vi "Sondenmodell.GetRef.vi"(8 "Error In":errorcluster) -> (0 "Error out":errorcluster, 3 "Sondenmodell":refnum<data-value>)   [LabVIEW 2016, in "Sondenmodell.lvclass"]
uses:
  Sondenmodell.lvclass
  Package ResourceControl/ObjectHandler/ObjectHandler.GetObjectWType.ctl
  Package ResourceControl/ObjectHandler/ObjectHandler.ObjectWType.ctl
  Package ResourceControl/ObjectHandler/ObjectHandler.ObjectType.ctl
  Package ResourceControl/ObjectHandler/ObjectHandler.lvclass
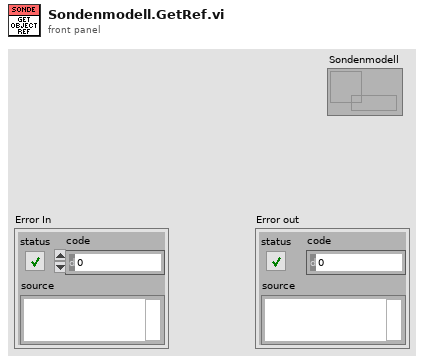
[diagram p1: front panel]
types:
  T1 = typedef "ObjectHandler.lvclass/ObjectHandler.GetObjectWType.ctl" = cluster{"Name":string, "Caller":string}
  T2 = typedef "ObjectHandler.lvclass/ObjectHandler.ObjectWType.ctl" = cluster{"ObjectType":T3, "Object":variant}
  T3 = typedef "ObjectHandler.lvclass/ObjectHandler.ObjectType.ctl" = enum16{"undefined", "ObjectHandler", "ViHandler", "ErrorHandler", "CentralStorage", "Hausmodell", "Sondenmodell", "Wärmepumpe", "Umgebung"}
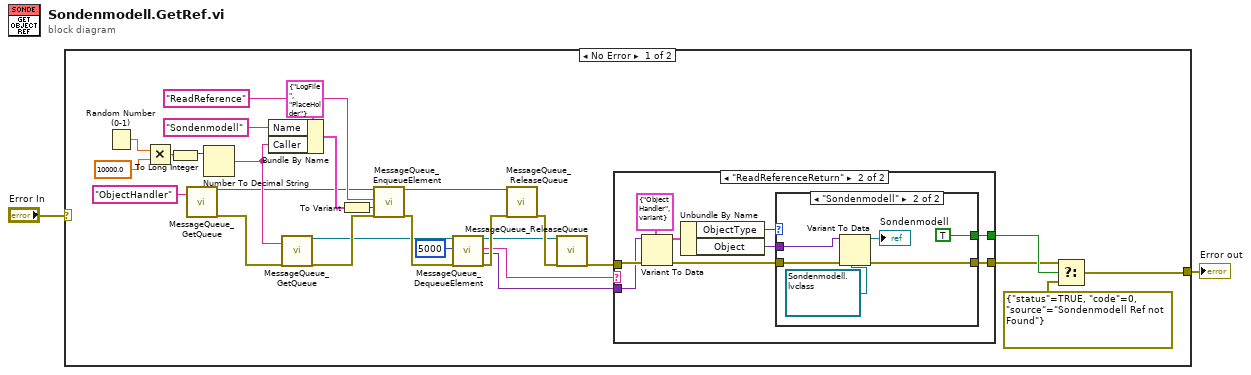
[diagram p0: block diagram]
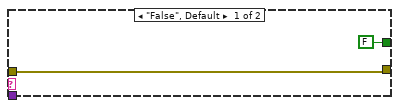
[diagram p2: hidden frame]
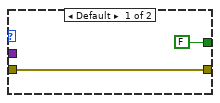
[diagram p3: hidden frame]
diagram:
  n1 = case shown="No Error" "Error In" {
    selector: "Error In" -> [_ w50]
    tunnel: [w30 w50] -> w2
    frame No Error {
      n2 = Random Number (0-1)() -> (number: 0 to 1=w29:dbl)
      n3 = Multiply(x=w29, y=10000.0) -> (x*y=w27:dbl)
      n4 = To Long Integer(number=w27) -> (32bit integer=w26:i32)
      n5 = call "MessageQueue_GetQueue.vi"("Name"="ObjectHandler") -> ("QueueOut"=w3:refnum<queue>, "ErrorOut"=w4:errorcluster)  [unwired: 16 in, 1 out]
      n6 = Number To Decimal String(number=w26) -> (decimal integer string=w11:string)  [unwired: 1 in]
      n7 = Bundle By Name(cluster=T1 {"Name"="LogFile", "Caller"="PlaceHolder"} ("GetRefInput"), "Name"="Sondenmodell", "Caller"=w11) -> (w10:T1)
      n8 = call "MessageQueue_GetQueue.vi"("Name"=w11, "ErrorIn"=w4) -> ("QueueOut"=w20:refnum<queue>, "ErrorOut"=w25:errorcluster)  [unwired: 15 in, 1 out]
      n9 = To Variant(anything=w10) -> (Variant=w15:variant)
      n10 = call "MessageQueue_EnqueueElement.vi"("QueueIn"=w3, "Message"="ReadReference", "Data"=w15, "ErrorIn"=w25) -> ("QueueOut"=w21:refnum<queue>, "ErrorOut"=w24:errorcluster)  [unwired: 14 in]
      n11 = call "MessageQueue_DequeueElement.vi"("QueueIn"=w20, "Timeout"=5000, "ErrorIn"=w24) -> ("QueueOut"=w19:refnum<queue>, "Message"=w17:string, "Data"=w13:variant, "ErrorOut"=w23:errorcluster)  [unwired: 12 in, 1 out]
      n12 = call "MessageQueue_ReleaseQueue.vi"("QueueIn"=w21, "ErrorIn"=w23) -> ("ErrorOut"=w22:errorcluster)  [unwired: 15 in, 2 out]
      n13 = call "MessageQueue_ReleaseQueue.vi"("QueueIn"=w19, "ErrorIn"=w22) -> ("ErrorOut"=w14:errorcluster)  [unwired: 15 in, 2 out]
      n14 = case shown="\"ReadReferenceReturn\"" w17 {
        tunnel: w14 -> [w31 w41]
        tunnel: w13 -> [_ w40]
        tunnel: [w31 w34] -> w8
        tunnel: [FALSE w33] -> w9
        frame "False", Default {
        }
        frame "ReadReferenceReturn" {
          n15 = Variant To Data(error in=w41, type=T2 {"ObjectType"=enum."ObjectHandler", "Object"=variant} ("ObjectWType"), Variant=w40) -> (data=w38:T2, error out=w35:errorcluster)
          n16 = Unbundle By Name(w38) -> ("ObjectType"=w37:T3, "Object"=w36:variant)
          n17 = case shown="\"Sondenmodell\"" w37 {
            tunnel: w36 -> [_ w49]
            tunnel: w35 -> [w43 w48]
            tunnel: [w43 w47] -> w34
            tunnel: [FALSE TRUE] -> w33
            frame Default {
            }
            frame "Sondenmodell" {
              n18 = Variant To Data(error in=w48, type=refnum<data-value> refnum ("data value reference"), Variant=w49) -> (data=→"Sondenmodell":refnum<data-value>, error out=w47:errorcluster)
            }
          }
        }
      }
      n19 = Select(t=w8, s=w9, f=errorcluster {"status"=TRUE, "code"=0, "source"="Sondenmodell Ref not Found"}) -> (s? t:f=w30:errorcluster)
    }
    frame Error {
    }
  }
  "Error out" <- w2
